vi "solar_qtimer Launch.vi"(6 "Suppress Errors? (T)":bool=TRUE, 7 "Open FP? (F)":bool, 8 "error in (no error)":errorcluster, 9 "Target Queue":refnum<queue>, 10 "QTimer Name":string, 11 "QTimer Refnum in":T1) -> (0 "error out":errorcluster, 3 "QTimer Refnum out":T1)   [LabVIEW 2018]
doc: "This launches a QTimer daemon to periodically enqueue messages to the target queue."
uses:
  solar_qtimer_ctl QTimer.ctl
  solar_qtimer_ctl QTimer Settings.ctl
  solar_qtimer_ctl Refnum.ctl
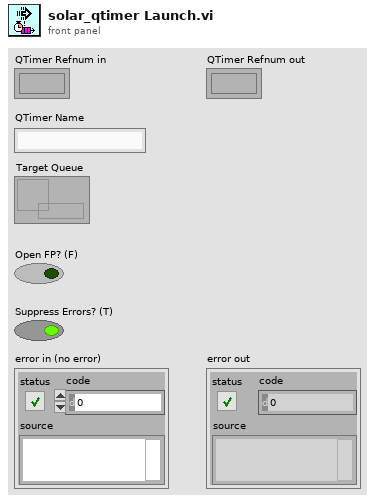
[diagram p1: front panel]
types:
  T1 = typedef "solar_qtimer_ctl Refnum.ctl" = refnum<k1>
  T2 = typedef "solar_qtimer_ctl QTimer.ctl" = cluster{"Settings":T3, "Queue":refnum<queue>, "QTimerQ":refnum<queue>, "VI Refnum":refnum<vi>}
  T3 = typedef "solar_qtimer_ctl QTimer Settings.ctl" = cluster{"QTimer":string, "Delay":i32, "Start":bool, "EnQ_Type":enum8{"Normal", "Priority", "IgnoreIfExists"}, "Messages":cluster{"MSG":string, "DATA":variant}[]}
  T4 = typedef "solar_qtimer_ctl SEQ.ctl" = cluster{"QTimers":T2[]}
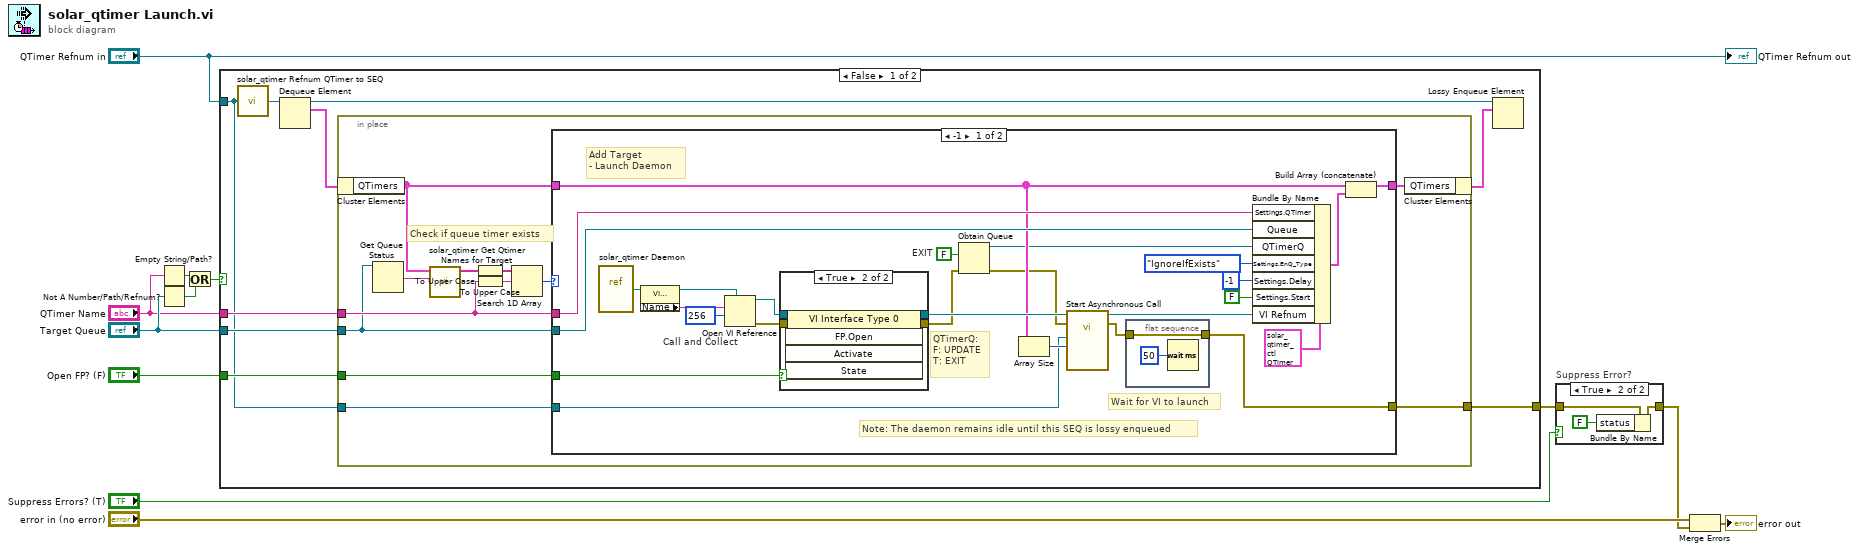
[diagram p0: block diagram]
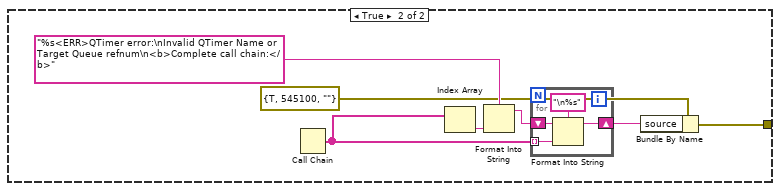
[diagram p4: hidden frame]
diagram:
  n1 = Empty String/Path?(string/path="QTimer Name") -> (empty?=w5:bool)
  n2 = Not A Number/Path/Refnum?(number/path/refnum="Target Queue") -> (NaN/Path/Refnum?=w4:bool)
  n3 = Or(x=w5, y=w4) -> (x .or. y?=w3:bool)
  n4 = case shown="False" w3 {
    tunnel: "QTimer Refnum in" -> [w14 _]
    tunnel: "QTimer Name" -> [w17 _]
    tunnel: "Target Queue" -> [w16 _]
    tunnel: [w13 w69] -> w2
    tunnel: "Open FP? (F)" -> [w15 _]
    frame False {
      n5 = call "solar_qtimer Refnum QTimer to SEQ.vi"("QTimer Refnum"=w14) -> ("QTimers SEQ"=w21:refnum<queue>)
      n6 = Dequeue Element(queue=w21) -> (queue out=w20:refnum<queue>, element=w19:T4)  [unwired: 2 in, 2 out]
      n7 = in-place {
        in-place-border: w17 -> [w26]
        in-place-border: w16 -> [w22]
        in-place-border: w15 -> [w27]
        in-place-border: [w25] -> w13
        in-place-border: w14 -> [w24]
        # "Check if queue timer exists"
        n8 = in-place-cluster #1(w19) -> ("QTimers"=w29:T2[])
        n9 = Get Queue Status(queue=w22) -> (queue name=w23:string)  [unwired: 2 in, 7 out]
        n10 = call "solar_qtimer Get Qtimer Names for Target.vi"("Target Name"=w23, "QTimers"=w29) -> ("Target's Qtimer Names"=w33:string[])  [unwired: 9 in]
        n11 = To Upper Case(1:w33) -> (0:w32:string[])
        n12 = To Upper Case(1:w26) -> (0:w31:string)
        n13 = Search 1D Array(1D array=w32, element=w31) -> (index of element=w30:i32)  [unwired: 1 in]
        n14 = case shown="-1" w30 {
          tunnel: w29 -> [w43 w68]
          tunnel: [w59 w68] -> w28
          tunnel: w27 -> [w48 _]
          tunnel: w26 -> [w47 _]
          tunnel: w22 -> [w46 _]
          tunnel: [w38 _] -> w25
          tunnel: w24 -> [w40 _]
          frame -1 {
            w55 = 256  # Call and Collect
            w37 = FALSE  # EXIT
            # "Wait for VI to launch"
            # "Note: The daemon remains idle until this SEQ is lossy enqueued"
            # "QTimerQ:\nF: UPDATE\nT: EXIT"
            # "Add Target\n- Launch Daemon"
            n15 = vi-ref "solar_qtimer Daemon.vi"() -> (w58:refnum<vi>)
            n16 = property class="VI (strict)"(reference=w58) -> (reference out=w56:refnum<vi>, "Name"=w57:string)  [unwired: 1 in, 1 out]
            n17 = Open VI Reference(type specifier VI Refnum (for type only)=w56, vi path=w57, options=w55) -> (vi reference=w53:refnum<vi>, error out=w54:errorcluster)  [unwired: 3 in]
            n18 = case shown="True" w48 {
              tunnel: w54 -> [w63 w67]
              tunnel: [w63 w66] -> w36
              tunnel: w53 -> [w62 w65]
              tunnel: [w62 w64] -> w44
              frame False {
              }
              frame True {
                n19 = invoke class="VI Interface Type 0" method="FP.Open"(reference=w65, error in=w67) -> (reference out=w64:refnum<vi>, error out=w66:errorcluster)  [unwired: 3 in, 3 out]
              }
            }
            n20 = Obtain Queue(element data type=w37, error in (no error)=w36) -> (queue out=w35:refnum<queue>, error out=w34:errorcluster)  [unwired: 3 in, 1 out]
            n21 = Array Size(array=w43) -> (size(s)=w42:i32)
            n22 = call-by-ref "Start Asynchronous Call"(reference=w44, error in=w34, "Instance"=w42, "QTimerRefnum"=w40) -> (reference out=w45:refnum<vi>, error out=w39:errorcluster)  [unwired: 9 in, 1 out]
            n23 = flat-sequence {
              tunnel: [w60] -> w38
              tunnel: w39 -> [w60]
              frame #0 {
                n24 = Wait (ms)(milliseconds to wait=u32 50) -> ()  [unwired: 1 out]
              }
            }
            n25 = Bundle By Name(cluster=T2 {"Settings"={"QTimer"="", "Delay"=0, "Start"=FALSE, "EnQ_Type"=enum."Normal", "Messages"=[]}, "Queue"=refnum, "QTimerQ"=refnum, "VI Refnum"=refnum} ("QTimer"), "Settings.QTimer"=w47, "Queue"=w46, "QTimerQ"=w35, "Settings.EnQ_Type"=enum8{"Normal", "Priority", "IgnoreIfExists"}."IgnoreIfExists" ("EnQ_Type"), "Settings.Delay"=-1 ("Delay"), "Settings.Start"=FALSE ("Running"), "VI Refnum"=w45) -> (w49:T2)
            n26 = Build Array (concatenate)(w43, w49) -> (w59:T2[])
          }
          frame Default {
            # "Already exists\n-Do nothing"
          }
        }
        n27 = in-place-cluster #1("QTimers"=w28) -> (w18:T4)
      }
      n28 = Lossy Enqueue Element(queue=w20, element=w18) -> ()  [unwired: 1 in, 4 out]
    }
    frame True {
      n29 = Call Chain() -> (call chain=w72:string[])
      n30 = Index Array(array=w72) -> (element=w74:string)  [unwired: 1 in]
      n31 = Format Into String(format string="%s<ERR>QTimer error:\nInvalid QTimer Name or Target Queue refnum\n<b>Complete call chain:</b>", w74) -> (resulting string=w73:string)  [unwired: 2 in, 1 out]
      n32 = for {
        tunnel: w72 -> [w79] mode=indexing
        shift-right: [w78] -> w71
        shift-left: w73 -> [w77]
        n33 = Format Into String(format string="\n%s", initial string=w77, w79) -> (resulting string=w78:string)  [unwired: 1 in, 1 out]
      }
      n34 = Bundle By Name(cluster=errorcluster {"status"=TRUE, "code"=545100, "source"=""} ("error in (no error)"), "source"=w71) -> (w69:errorcluster)
    }
  }
  n35 = case "Suppress Error?" shown="True" "Suppress Errors? (T)" {
    tunnel: w2 -> [w80 w83]
    tunnel: [w80 w82] -> w8
    frame False {
    }
    frame True {
      n36 = Bundle By Name(cluster=w83, "status"=FALSE) -> (w82:errorcluster)
    }
  }
  n37 = Merge Errors("error in (no error)", w8) -> (→"error out":errorcluster)
  "QTimer Refnum out" <- "QTimer Refnum in"
